vi "PWM SubVI.vi"(0 "error in (no error)":errorcluster, 1 "PWM Frequency":dbl(slide) scale=10.0..10000.0, 5 "Motor 1 Duty Cycle":dbl(slide) scale=0.0..1.0, 7 "Motor 2 Duty Cycle":dbl(slide) scale=0.0..1.0, 9 "Motor 3 Duty Cycle":dbl(slide) scale=0.0..1.0, 11 "Motor 4 Duty Cycle":dbl(slide) scale=0.0..1.0) -> (4 "error out":errorcluster)   [LabVIEW 2014]
uses:
  <vilib>/myRIO/Instrument Drivers/Onboard IO/PWM/typedefs/PWM Reference.ctl
  <vilib>/myRIO/Common/Instrument Driver Framework/Utilities/typedefs/myRIO Generic Hardware Reference.ctl
  <vilib>/myRIO/Common/Instrument Driver Framework/Utilities/typedefs/Hardware Version Enum.ctl
  <vilib>/myRIO/Common/Instrument Driver Framework/Utilities/typedefs/myRIO v1.0 Reference.ctl
  <vilib>/myRIO/Common/Instrument Driver Framework/Utilities/typedefs/Generic FPGA Reference.ctl
  <vilib>/myRIO/Common/Instrument Driver Framework/myRIO v1.0/PWM/typedefs/PWM Channels Enum.ctl
  <vilib>/myRIO/Instrument Drivers/Onboard IO/PWM/typedefs/PWM Configuration.ctl
  <vilib>/userdefined/High Color/nirio_resource_hc.ctl
  <vilib>/myRIO/Common/Instrument Driver Framework/Utilities/vis/Is FPGA Ref Available.vi
  <vilib>/myRIO/Common/Instrument Driver Framework/myRIO v1.0/PWM/vis/myRIO v1.1 Open PWM.vi
  <vilib>/myRIO/Instrument Drivers/Onboard IO/PWM/vis/Set Duty Cycle and Frequency.vi
  <vilib>/myRIO/Common/Instrument Driver Framework/Utilities/vis/Validate Channels.vi
  <vilib>/myRIO/Common/Instrument Driver Framework/myRIO v1.0/PWM/vis/myRIO v1.0 Reserve PWM.vi
  <vilib>/myRIO/Common/Instrument Driver Framework/myRIO v1.0/PWM/vis/myRIO v1.0 Build MUX Configuration PWM.vi
  <vilib>/myRIO/Common/Instrument Driver Framework/myRIO v1.0/Resource Manager/vis/myRIO v1.0 Reserve Channel List.vi
  <vilib>/myRIO/Common/Instrument Driver Framework/myRIO v1.0/Resource Manager/vis/myRIO v1.0 Create Configuration List.vi
  <vilib>/myRIO/Common/Instrument Driver Framework/myRIO v1.0/Resource Manager/vis/myRIO v1.0 Reserve Channel.vi
  <vilib>/myRIO/Common/Instrument Driver Framework/myRIO v1.0/Resource Manager/vis/myRIO v1.0 Unreserve Channel.vi
  <vilib>/myRIO/Common/Instrument Driver Framework/myRIO v1.0/Resource Manager/vis/myRIO v1.0 Build Mutex Name.vi
  <vilib>/myRIO/Instrument Drivers/Onboard IO/PWM/vis/Smart Open.vi
  <vilib>/Utility/error.llb/Error Cluster From Error Code.vi
  <vilib>/myRIO/Common/Instrument Driver Framework/myRIO v1.0/PWM/vis/myRIO v1.0 Write PWM.vi
  <vilib>/Utility/VariantDataType/GetNumericInfo.vi
  <vilib>/myRIO/Common/Instrument Driver Framework/myRIO v1.0/myRIO v1.1 Open.vi
  <vilib>/myRIO/Common/Instrument Driver Framework/Utilities/vis/IO Manager.vi
  <vilib>/myRIO/Common/Instrument Driver Framework/Utilities/vis/Configuration Manager.vi
  <vilib>/myRIO/Common/Instrument Driver Framework/myRIO v1.0/Resource Manager/vis/myRIO v1.0 Configure IO.vi
  <vilib>/myRIO/Common/Instrument Driver Framework/myRIO v1.0/myRIO v1.0 Close.vi
  <vilib>/myRIO/Express VI/Onboard IO/PWM/PWM Express VI.xnode
  <vilib>/myRIO/Instrument Drivers/Onboard IO/PWM/vis/myRIO PWM Open.xnode
  <vilib>/myRIO/Instrument Drivers/Onboard IO/PWM/PWM.lvlib
panel:
  # "This SubVI just controls the 4 PWM Channels on the buggy\nThey are all coming out of connectors A and B"
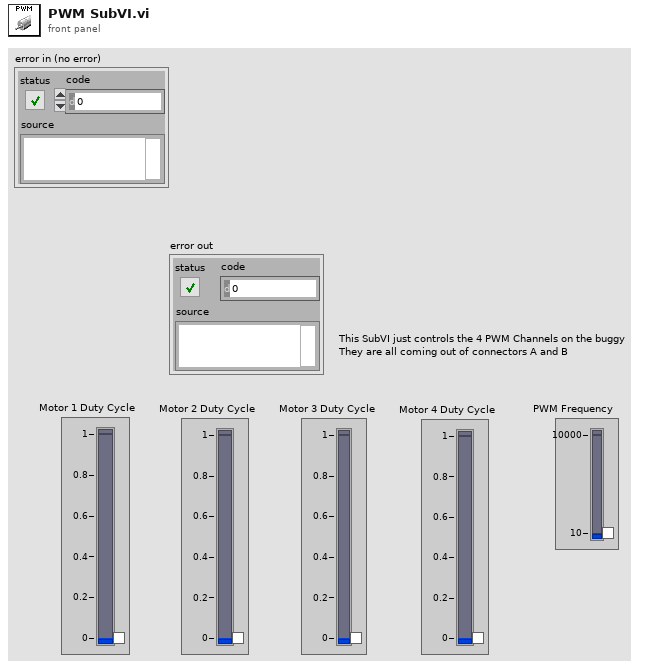
[diagram p1: front panel]
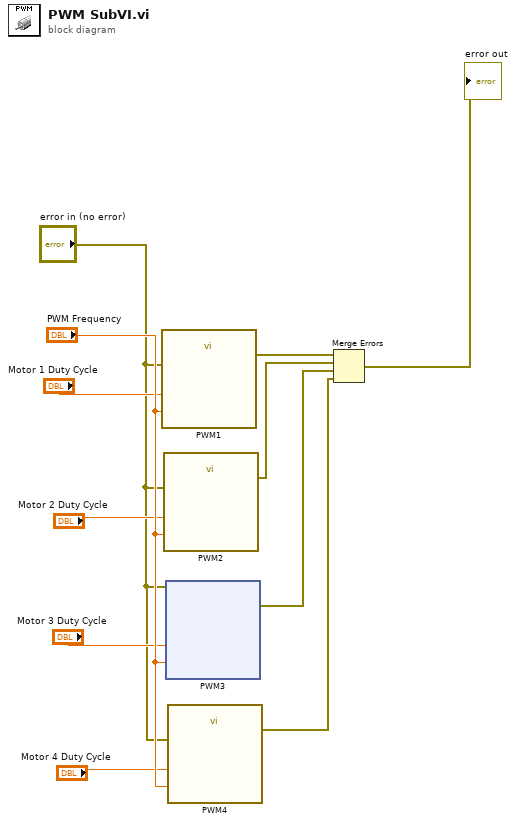
[diagram p0: block diagram]
diagram:
  n1 = call "PWM1"("Duty Cycle (0-1)"="Motor 1 Duty Cycle", "Frequency (Hz)"="PWM Frequency", "error in (no error)"="error in (no error)") -> ("error out"=w6:errorcluster)  [unwired: 24 in]
  n2 = call "PWM2"("Duty Cycle (0-1)"="Motor 2 Duty Cycle", "Frequency (Hz)"="PWM Frequency", "error in (no error)"="error in (no error)") -> ("error out"=w7:errorcluster)  [unwired: 24 in]
  n3 = xnode "PWM3"("Duty Cycle"="Motor 3 Duty Cycle", "Frequency [Hz]"="PWM Frequency", "error in (no error)"="error in (no error)") -> ("error out"=w8:errorcluster)
  n4 = call "PWM4"("Duty Cycle (0-1)"="Motor 4 Duty Cycle", "Frequency (Hz)"="PWM Frequency", "error in (no error)"="error in (no error)") -> ("error out"=w9:errorcluster)  [unwired: 24 in]
  n5 = Merge Errors(w6, w7, w8, w9) -> (→"error out":errorcluster)
